vi "certaintyGraph.vi"(8 "Detected":bool, 9 "Y":u16, 10 "X":i16, 11 "Array":i16[][](array[numeric])) -> (3 "Array 2":i16[][](array[numeric]))   [LabVIEW 2012]
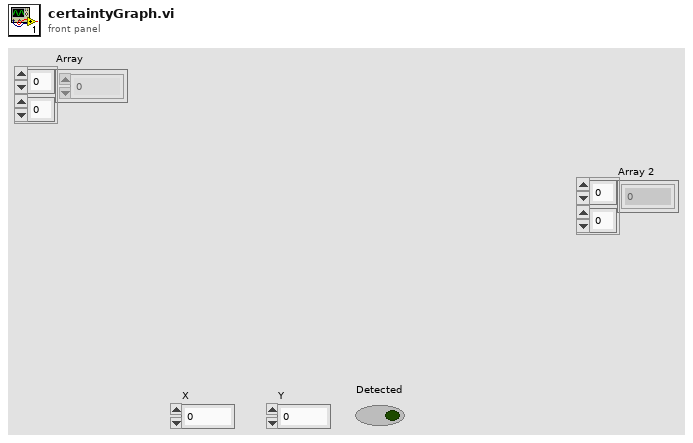
[diagram p1: front panel]
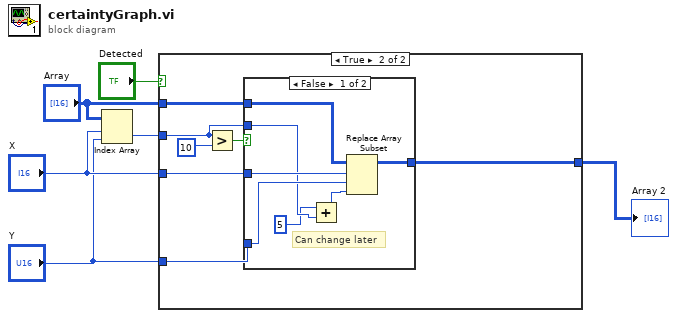
[diagram p0: block diagram]
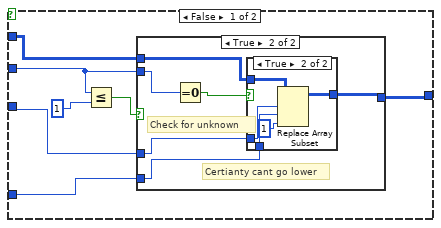
[diagram p2: hidden frame]
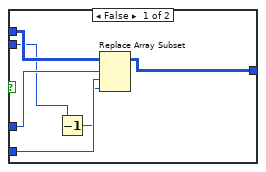
[diagram p3: hidden frame]
diagram:
  n1 = Index Array(array="Array", index (row)="X", index (col)="Y") -> (element=w5:i16)
  n2 = case shown="True" "Detected" {
    tunnel: w5 -> [w11 w33]
    tunnel: "Array" -> [w10 w38]
    tunnel: "X" -> [w9 w37]
    tunnel: "Y" -> [w8 w36]
    tunnel: [w7 w32] -> w1
    frame False {
      n3 = Less Or Equal?(x=w11, y=1) -> (x <= y?=w12:bool)
      n4 = case shown="True" w12 {
        tunnel: w11 -> [w15 w24]
        tunnel: w10 -> [w19 w23]
        tunnel: w9 -> [w17 w21]
        tunnel: w8 -> [w16 w20]
        tunnel: [w18 w22] -> w7
        frame False {
          n5 = Decrement(x=w15) -> (x-1=w14:i16)
          n6 = Replace Array Subset(array=w19, new element=w14, index (row)=w17, index (col)=w16) -> (w18:i16[][])
        }
        frame True {
          # "Check for unknown"
          # "Certianty cant go lower"
          n7 = Equal To 0?(x=w24) -> (x = 0?=w25:bool)
          n8 = case shown="True" w25 {
            tunnel: w23 -> [w26 w31]
            tunnel: [w26 w30] -> w22
            tunnel: w21 -> [_ w29]
            tunnel: w20 -> [_ w28]
            frame False {
            }
            frame True {
              n9 = Replace Array Subset(array=w31, new element=1, index (row)=w29, index (col)=w28) -> (w30:i16[][])
            }
          }
        }
      }
    }
    frame True {
      n10 = Greater?(x=w33, y=10) -> (0:w34:bool)
      n11 = case shown="False" w34 {
        tunnel: w38 -> [w43 w46]
        tunnel: w37 -> [w45 _]
        tunnel: w36 -> [w44 _]
        tunnel: w33 -> [w41 _]
        tunnel: [w42 w46] -> w32
        frame False {
          # "Can change later"
          n12 = Add(x=i16 5, y=w41) -> (x+y=w40:i16)
          n13 = Replace Array Subset(array=w43, new element=w40, index (row)=w45, index (col)=w44) -> (w42:i16[][])
        }
        frame True {
          # "Certainty cant go higher"
        }
      }
    }
  }
  "Array 2" <- w1
